vi "采水流程.vi"(10 "启动类型":enum16{"水样测试", "加标回收"}(ring), 11 "采配水参数":T1={"排空时间"=60.0, "润洗时间"=60.0, "进样超时时间"=300.0, "沉淀时间"=1800.0, "配水时间"=7200.0}) -> ()   [LabVIEW 2016, in "采配水.lvlib"]
panel:
  out "配水启动时间":timestamp
  in  "沉淀初始化":bool
  in  "配水初始化":bool
  in  "润洗初始化":bool
  in  "采样初始化":bool
  in  "排空初始化":bool
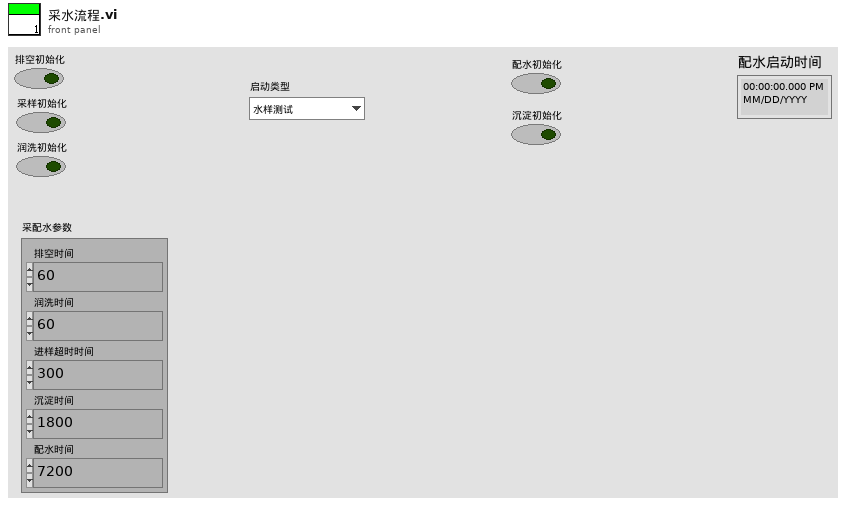
[diagram p1: front panel]
types:
  T1 = cluster{"排空时间":dbl, "润洗时间":dbl, "进样超时时间":dbl, "沉淀时间":dbl, "配水时间":dbl}
  T2 = typedef "采配水.lvlib/采配水流程.ctl" = u16
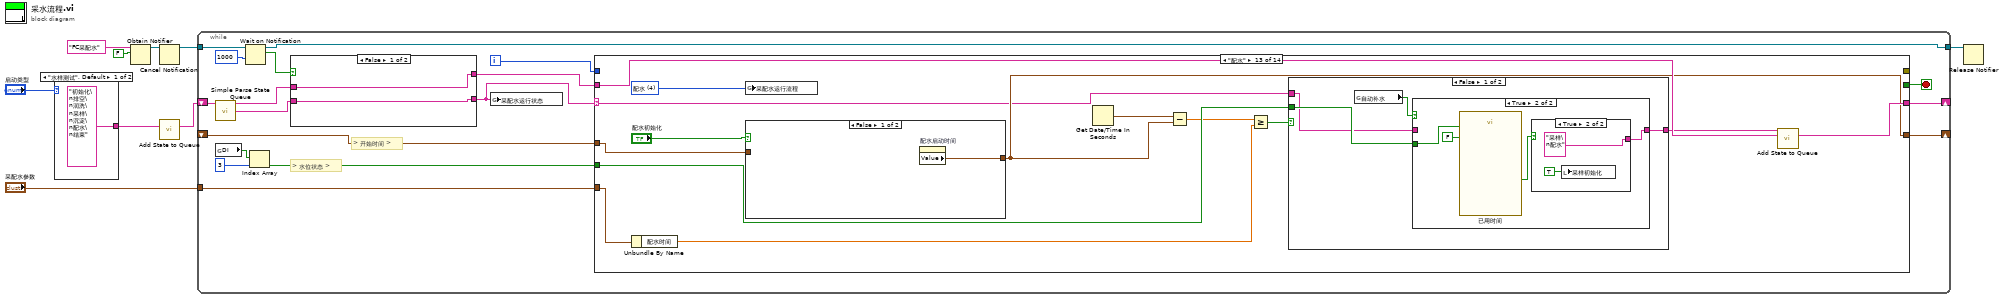
[diagram p0: block diagram]
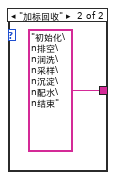
[diagram p2: hidden frame]
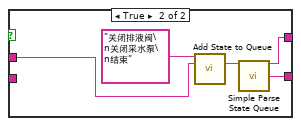
[diagram p3: hidden frame]
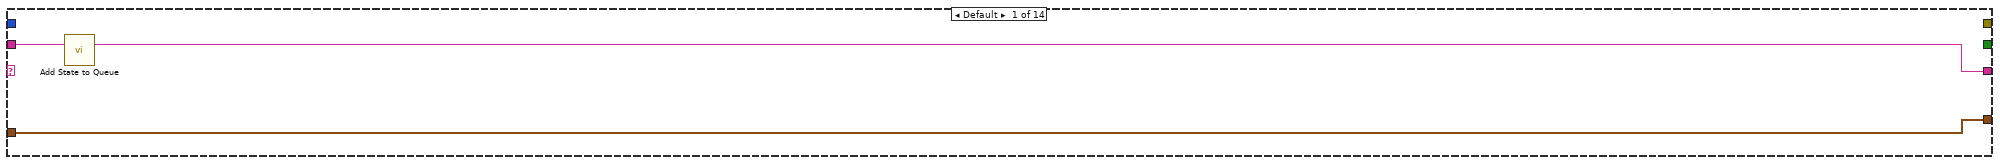
[diagram p4: hidden frame]
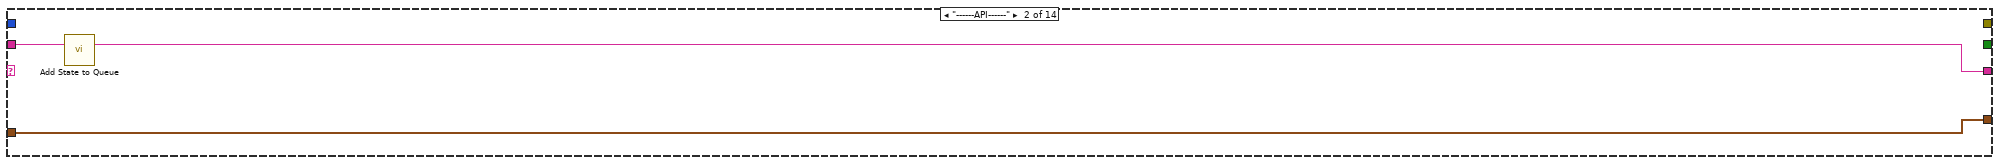
[diagram p5: hidden frame]
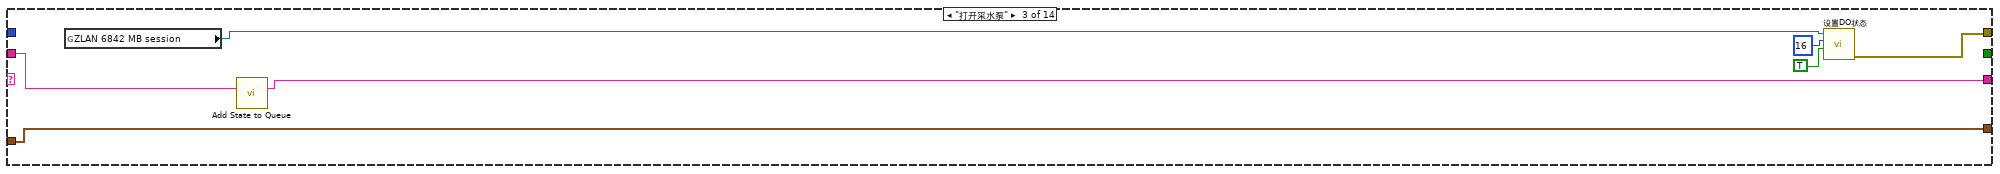
[diagram p6: hidden frame]
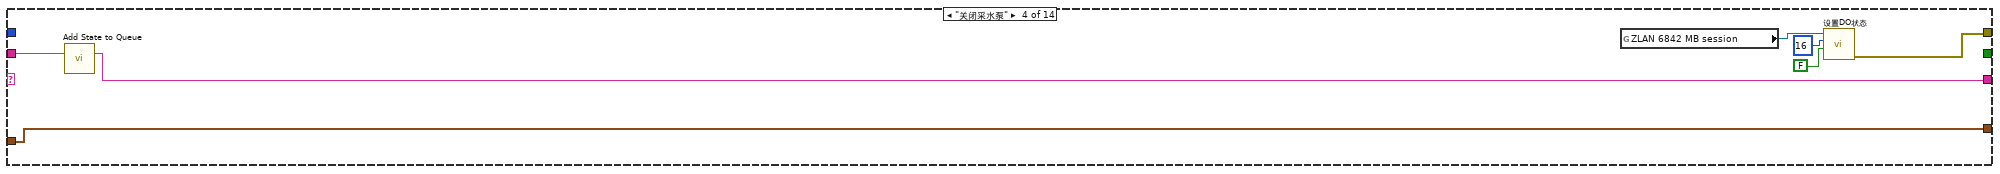
[diagram p7: hidden frame]
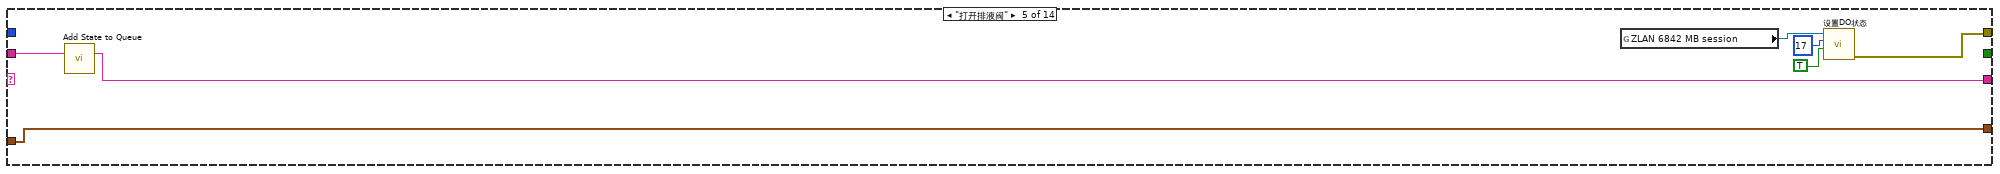
[diagram p8: hidden frame]
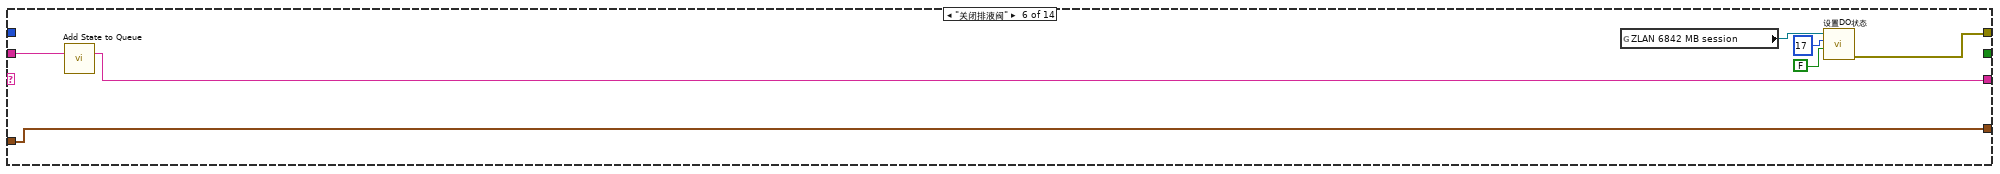
[diagram p9: hidden frame]
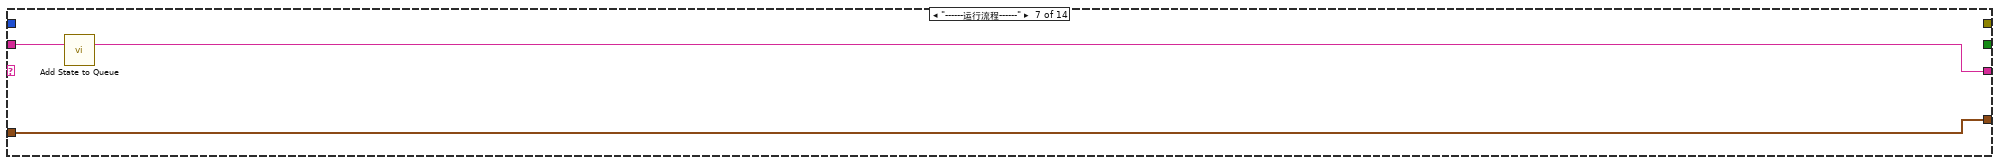
[diagram p10: hidden frame]
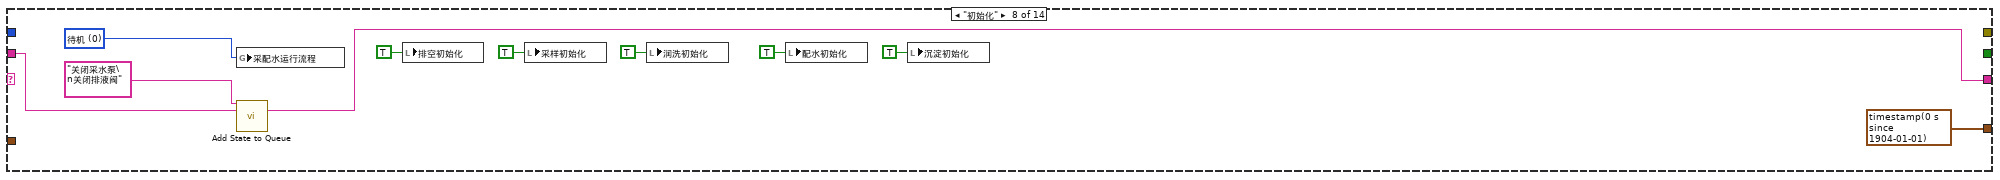
[diagram p11: hidden frame]
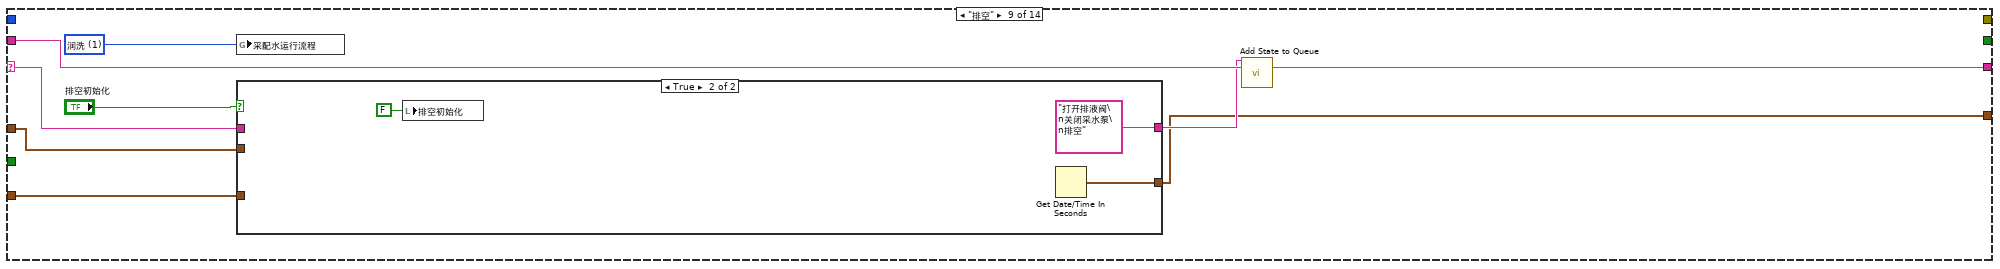
[diagram p12: hidden frame]
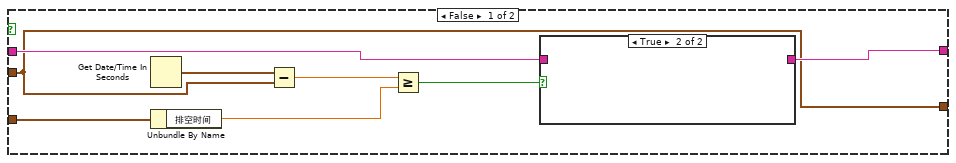
[diagram p13: hidden frame]
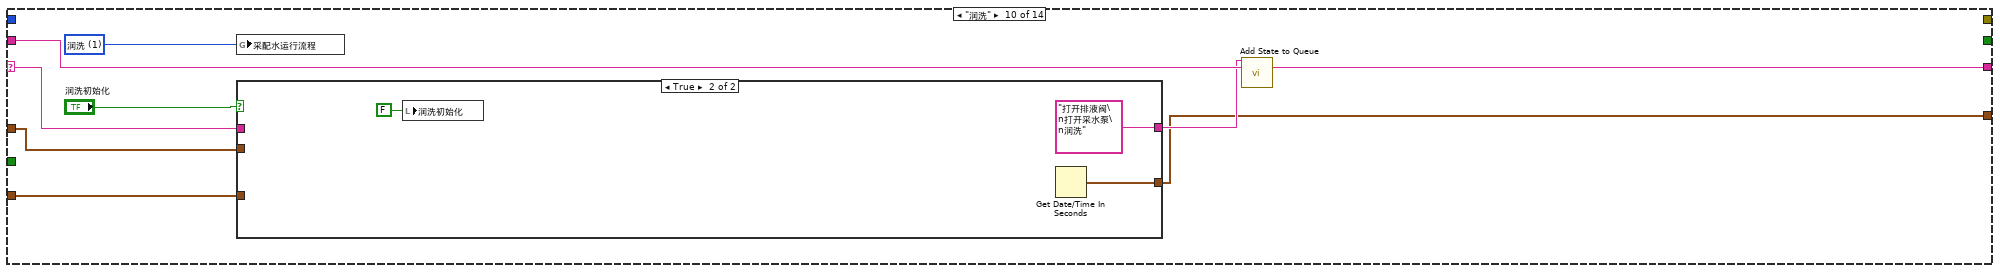
[diagram p15: hidden frame]
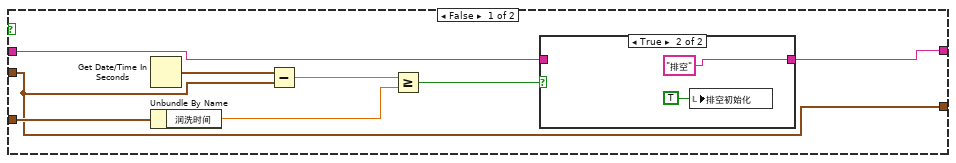
[diagram p16: hidden frame]
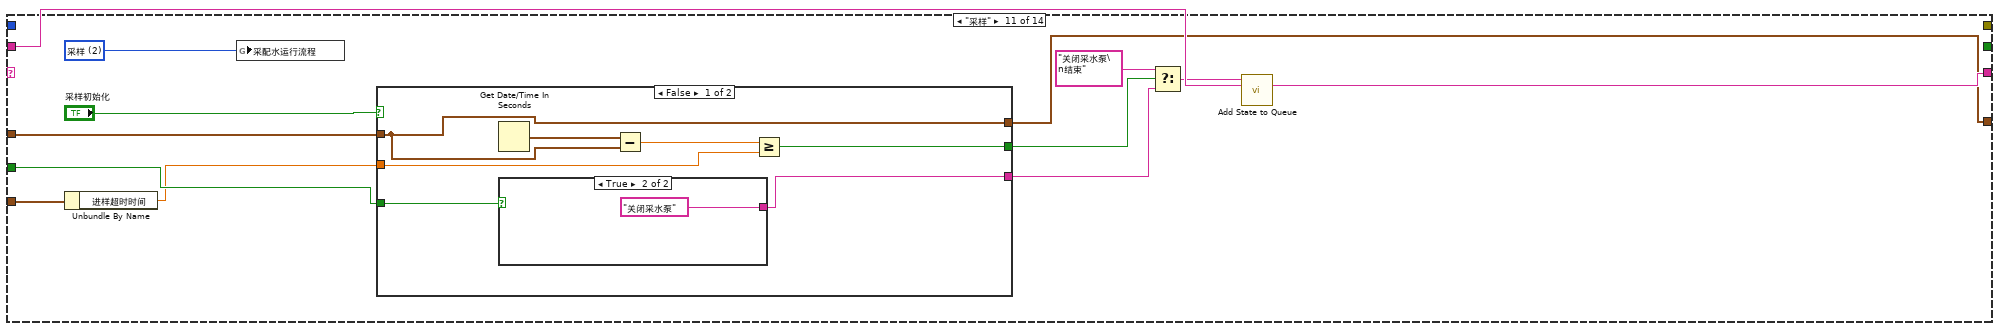
[diagram p18: hidden frame]
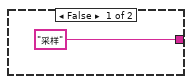
[diagram p19: hidden frame]
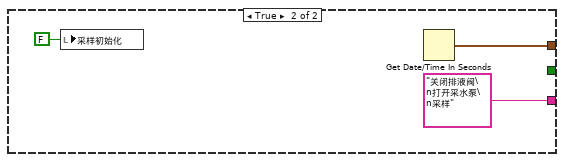
[diagram p20: hidden frame]
diagram:
  n1 = case shown="\"水样测试\", Default" "启动类型" {
    tunnel: ["初始化\n排空\n润洗\n采样\n沉淀\n配水\n结束" ("State(s) In (\"\")") "初始化\n排空\n润洗\n采样\n沉淀\n配水\n结束" ("State(s) In (\"\")")] -> w2
    frame "水样测试", Default {
    }
    frame "加标回收" {
    }
  }
  n2 = Obtain Notifier(name (unnamed)="FC采配水" ("名称（未命名）"), notification data type=FALSE) -> (notifier out=w6:refnum<notifier>)  [unwired: 2 in, 2 out]
  n3 = Cancel Notification(0:w6) -> (8:w5:refnum<notifier>)  [unwired: 1 in, 2 out]
  n4 = call "Add State to Queue.vi"("State(s) In (\"\")"=w2) -> ("States Out"=w9:string)  [unwired: 14 in]
  n5 = while {
    shift-right: [w28] -> _
    shift-left: w9 -> [w29]
    shift-right: [w27] -> _
    shift-left: _ -> [w26]
    tunnel: "采配水参数" -> [w21]
    tunnel: w5 -> [w20]
    tunnel: [w16] -> w4
    i -> [w12]
    stop <- w25 stop-if-true
    # "> 开始时间 >"
    # "> 水位状态 >"
    n6 = call "Simple Parse State Queue.vi"("State Queue"=w29) -> ("Remain States"=w15:string, "Next State"=w17:string)  [unwired: 13 in]
    n7 = global read "通讯全局变量.vi" "DI"() -> (w24:bool[])
    n8 = Wait on Notification(notifier=w20, timeout in ms (-1)=1000 ("超时毫秒(-1)")) -> (notifier out=w16:refnum<notifier>, notification=w18:bool)  [unwired: 2 in, 2 out]
    n9 = Index Array(array=w24, index=3 ("索引")) -> (element=w22:bool)
    n10 = case shown="False" w18 {
      tunnel: [w31 w33] -> w13
      tunnel: w17 -> [w31 _]
      tunnel: w15 -> [w30 w35]
      tunnel: [w30 w32] -> w14
      frame False {
      }
      frame True {
        n11 = call "Add State to Queue.vi"("State(s) In Front (\"\")"="关闭排液阀\n关闭采水泵\n结束" ("State(s) In (\"\")"), "State(s) In (\"\")"=w35) -> ("States Out"=w34:string)  [unwired: 13 in]
        n12 = call "Simple Parse State Queue.vi"("State Queue"=w34) -> ("Remain States"=w32:string, "Next State"=w33:string)  [unwired: 13 in]
      }
    }
    n13 = global write "通讯全局变量.vi" "采配水运行状态"(w13) -> ()
    n14 = case shown="\"配水\"" w13 {
      selector: w13 -> [_ _ _ _ _ _ _ _ w89 w109 _ w153 w170 w199]
      tunnel: w14 -> [w39 w42 w49 w56 w63 w70 w73 w83 w92 w111 w140 w160 w180 _]
      tunnel: [w38 w41 w48 w55 w62 w69 w72 w82 w91 w113 w139 w165 w183 w199] -> w28
      tunnel: w22 -> [_ _ _ _ _ _ _ _ _ _ w138 _ w182 _]
      tunnel: [_ _ w44 w51 w58 w65 _ _ _ _ _ _ _ _] -> _
      tunnel: [w37 w40 w43 w50 w57 w64 w71 timestamp(0 s since 1904-01-01) ("seconds since 1Jan1904") w84 w105 w128 w155 w174 w202] -> w27
      tunnel: w26 -> [w37 w40 w43 w50 w57 w64 w71 _ w90 w112 w133 w157 w176 w202]
      tunnel: [_ _ _ _ _ _ _ _ _ _ _ _ _ TRUE] -> w25
      tunnel: w21 -> [_ _ _ _ _ _ _ _ w86 w108 w137 w163 w179 _]
      tunnel: w12 -> [_ _ _ _ _ _ _ _ _ _ _ _ _ _]
      frame Default {
        n15 = call "Add State to Queue.vi"("State(s) In (\"\")"=w39) -> ("States Out"=w38:string)  [unwired: 14 in]
      }
      frame "------API------" {
        n16 = call "Add State to Queue.vi"("State(s) In (\"\")"=w42) -> ("States Out"=w41:string)  [unwired: 14 in]
      }
      frame "打开采水泵" {
        n17 = global read "通讯全局变量.vi" "ZLAN 6842 MB session"() -> (w45:refnum<class "MB_Master.lvclass">)
        n18 = call "Add State to Queue.vi"("State(s) In (\"\")"=w49) -> ("States Out"=w48:string)  [unwired: 14 in]
        n19 = call "设置DO状态.vi"("value"=TRUE, "address"=u16 16, "MB session in"=w45) -> ("error out"=w44:errorcluster)  [unwired: 7 in, 1 out]
      }
      frame "关闭采水泵" {
        n20 = call "Add State to Queue.vi"("State(s) In (\"\")"=w56) -> ("States Out"=w55:string)  [unwired: 14 in]
        n21 = global read "通讯全局变量.vi" "ZLAN 6842 MB session"() -> (w52:refnum<class "MB_Master.lvclass">)
        n22 = call "设置DO状态.vi"("value"=FALSE, "address"=u16 16, "MB session in"=w52) -> ("error out"=w51:errorcluster)  [unwired: 7 in, 1 out]
      }
      frame "打开排液阀" {
        n23 = call "Add State to Queue.vi"("State(s) In (\"\")"=w63) -> ("States Out"=w62:string)  [unwired: 14 in]
        n24 = global read "通讯全局变量.vi" "ZLAN 6842 MB session"() -> (w59:refnum<class "MB_Master.lvclass">)
        n25 = call "设置DO状态.vi"("value"=TRUE, "address"=u16 17, "MB session in"=w59) -> ("error out"=w58:errorcluster)  [unwired: 7 in, 1 out]
      }
      frame "关闭排液阀" {
        n26 = call "Add State to Queue.vi"("State(s) In (\"\")"=w70) -> ("States Out"=w69:string)  [unwired: 14 in]
        n27 = global read "通讯全局变量.vi" "ZLAN 6842 MB session"() -> (w66:refnum<class "MB_Master.lvclass">)
        n28 = call "设置DO状态.vi"("value"=FALSE, "address"=u16 17, "MB session in"=w66) -> ("error out"=w65:errorcluster)  [unwired: 7 in, 1 out]
      }
      frame "------运行流程------" {
        n29 = call "Add State to Queue.vi"("State(s) In (\"\")"=w73) -> ("States Out"=w72:string)  [unwired: 14 in]
      }
      frame "初始化" {
        w76 = T2 0 items=["待机", "润洗", "采样", "沉淀", "配水", "结束"] ("采配水运行流程")
        n30 = global write "通讯全局变量.vi" "采配水运行流程"(w76) -> ()
        n31 = call "Add State to Queue.vi"("State(s) In Front (\"\")"="关闭采水泵\n关闭排液阀" ("State(s) In Front (\"\")"), "State(s) In (\"\")"=w83) -> ("States Out"=w82:string)  [unwired: 13 in]
        n32 = local write "排空初始化"(TRUE ("排空初始化")) -> ()
        n33 = local write "采样初始化"(TRUE ("采样初始化")) -> ()
        n34 = local write "润洗初始化"(TRUE ("润洗初始化")) -> ()
        n35 = local write "配水初始化"(TRUE ("采样初始化")) -> ()
        n36 = local write "沉淀初始化"(TRUE ("润洗初始化")) -> ()
      }
      frame "排空" {
        w85 = T2 1 items=["待机", "润洗", "采样", "沉淀", "配水", "结束"] ("采配水运行流程")
        n37 = global write "通讯全局变量.vi" "采配水运行流程"(w85) -> ()
        n38 = case shown="True" "排空初始化" {
          tunnel: [w97 "打开排液阀\n关闭采水泵\n排空" ("State(s) In Front (\"\")")] -> w88
          tunnel: w90 -> [w93 _]
          tunnel: w89 -> [w96 _]
          tunnel: w86 -> [w95 _]
          tunnel: [w93 w102] -> w84
          frame False {
            n39 = Get Date/Time In Seconds() -> (seconds since 1Jan1904=w98:timestamp)
            n40 = Unbundle By Name(w95) -> ("排空时间"=w94:dbl)
            n41 = Subtract(x=w98, y=w93) -> (x-y=w99:dbl)
            n42 = Greater Or Equal?(x=w99, y=w94) -> (x >= y?=w100:bool)
            n43 = case shown="True" w100 {
              tunnel: [w101 _] -> w97
              tunnel: w96 -> [w101 _]
              frame False {
              }
              frame True {
              }
            }
          }
          frame True {
            n44 = local write "排空初始化"(FALSE ("排空初始化")) -> ()
            n45 = Get Date/Time In Seconds() -> (seconds since 1Jan1904=w102:timestamp)
          }
        }
        n46 = call "Add State to Queue.vi"("State(s) In Front (\"\")"=w88, "State(s) In (\"\")"=w92) -> ("States Out"=w91:string)  [unwired: 13 in]
      }
      frame "润洗" {
        w106 = T2 1 items=["待机", "润洗", "采样", "沉淀", "配水", "结束"] ("采配水运行流程")
        n47 = global write "通讯全局变量.vi" "采配水运行流程"(w106) -> ()
        n48 = case shown="True" "润洗初始化" {
          tunnel: [w118 "打开排液阀\n打开采水泵\n润洗" ("State(s) In Front (\"\")")] -> w110
          tunnel: w112 -> [w114 _]
          tunnel: w109 -> [w117 _]
          tunnel: w108 -> [w116 _]
          tunnel: [w114 w125] -> w105
          frame False {
            n49 = Get Date/Time In Seconds() -> (seconds since 1Jan1904=w119:timestamp)
            n50 = Unbundle By Name(w116) -> ("润洗时间"=w115:dbl)
            n51 = Subtract(x=w119, y=w114) -> (x-y=w120:dbl)
            n52 = Greater Or Equal?(x=w120, y=w115) -> (x >= y?=w121:bool)
            n53 = case shown="True" w121 {
              tunnel: [w122 "排空"] -> w118
              tunnel: w117 -> [w122 _]
              frame False {
              }
              frame True {
                n54 = local write "排空初始化"(TRUE ("排空初始化")) -> ()
              }
            }
          }
          frame True {
            n55 = local write "润洗初始化"(FALSE ("润洗初始化")) -> ()
            n56 = Get Date/Time In Seconds() -> (seconds since 1Jan1904=w125:timestamp)
          }
        }
        n57 = call "Add State to Queue.vi"("State(s) In Front (\"\")"=w110, "State(s) In (\"\")"=w111) -> ("States Out"=w113:string)  [unwired: 13 in]
      }
      frame "采样" {
        w129 = T2 2 items=["待机", "润洗", "采样", "沉淀", "配水", "结束"] ("采配水运行流程")
        n58 = Unbundle By Name(w137) -> ("进样超时时间"=w132:dbl)
        n59 = global write "通讯全局变量.vi" "采配水运行流程"(w129) -> ()
        n60 = case shown="False" "采样初始化" {
          tunnel: [w146 "关闭排液阀\n打开采水泵\n采样" ("State(s) In Front (\"\")")] -> w136
          tunnel: w138 -> [w147 _]
          tunnel: w133 -> [w141 _]
          tunnel: w132 -> [w143 _]
          tunnel: [w142 _] -> w131
          tunnel: [w141 w150] -> w128
          frame False {
            n61 = Get Date/Time In Seconds() -> (seconds since 1Jan1904=w144:timestamp)
            n62 = case shown="True" w147 {
              tunnel: ["采样" ("State(s) In Front (\"\")") "关闭采水泵" ("State(s) In Front (\"\")")] -> w146
              frame False {
              }
              frame True {
              }
            }
            n63 = Subtract(x=w144, y=w141) -> (x-y=w145:dbl)
            n64 = Greater Or Equal?(x=w145, y=w143) -> (x >= y?=w142:bool)
          }
          frame True {
            n65 = local write "采样初始化"(FALSE ("采样初始化")) -> ()
            n66 = Get Date/Time In Seconds() -> (seconds since 1Jan1904=w150:timestamp)
          }
        }
        n67 = Select(t="关闭采水泵\n结束" ("State(s) In Front (\"\")"), s=w131, f=w136) -> (s? t:f=w135:string)
        n68 = call "Add State to Queue.vi"("State(s) In Front (\"\")"=w135, "State(s) In (\"\")"=w140) -> ("States Out"=w139:string)  [unwired: 13 in]
      }
      frame "沉淀" {
        w164 = T2 3 items=["待机", "润洗", "采样", "沉淀", "配水", "结束"] ("采配水运行流程")
        n69 = Unbundle By Name(w163) -> ("沉淀时间"=w162:dbl)
        n70 = global write "通讯全局变量.vi" "采配水运行流程"(w164) -> ()
        n71 = case shown="True" "沉淀初始化" {
          tunnel: w157 -> [w166 _]
          tunnel: [w166 w167] -> w155
          frame False {
          }
          frame True {
            n72 = property on="沉淀初始化" class="Bool (严格)"("Value"=FALSE ("沉淀初始化")) -> ()  [unwired: 2 in, 2 out]
            n73 = Get Date/Time In Seconds() -> (seconds since 1Jan1904=w167:timestamp)
          }
        }
        n74 = Get Date/Time In Seconds() -> (seconds since 1Jan1904=w156:timestamp)
        n75 = Subtract(x=w156, y=w155) -> (x-y=w154:dbl)
        n76 = Greater Or Equal?(x=w154, y=w162) -> (x >= y?=w161:bool)
        n77 = case shown="False" w161 {
          tunnel: [w169 _] -> w159
          tunnel: w153 -> [w169 _]
          frame False {
          }
          frame True {
          }
        }
        n78 = call "Add State to Queue.vi"("State(s) In Front (\"\")"=w159, "State(s) In (\"\")"=w160) -> ("States Out"=w165:string)  [unwired: 13 in]
      }
      frame "配水" {
        w181 = T2 4 items=["待机", "润洗", "采样", "沉淀", "配水", "结束"] ("采配水运行流程")
        n79 = Unbundle By Name(w179) -> ("配水时间"=w172:dbl)
        n80 = global write "通讯全局变量.vi" "采配水运行流程"(w181) -> ()
        n81 = case shown="False" "配水初始化" {
          tunnel: w176 -> [_ _]
          tunnel: [w196 w198] -> w174
          frame False {
            n82 = property on="配水启动时间" class="AbsTime (严格)"() -> ("Value"=w196:timestamp)  [unwired: 2 in, 2 out]
          }
          frame True {
            n83 = Get Date/Time In Seconds() -> (seconds since 1Jan1904=w198:timestamp)
            "配水启动时间" <- w198
            n84 = property on="配水初始化" class="Bool (严格)"("Value"=FALSE ("配水初始化")) -> ()  [unwired: 2 in, 2 out]
          }
        }
        n85 = Get Date/Time In Seconds() -> (seconds since 1Jan1904=w175:timestamp)
        n86 = Subtract(x=w175, y=w174) -> (x-y=w173:dbl)
        n87 = Greater Or Equal?(x=w173, y=w172) -> (x >= y?=w171:bool)
        n88 = case shown="False" w171 {
          tunnel: w182 -> [w187 _]
          tunnel: w170 -> [w185 _]
          tunnel: [w184 _] -> w178
          frame False {
            n89 = global read "通讯全局变量断电保存.vi" "自动补水"() -> (w186:bool)
            n90 = case shown="True" w186 {
              tunnel: w187 -> [_ w191]
              tunnel: [w188 w189] -> w184
              tunnel: w185 -> [w188 _]
              frame False {
              }
              frame True {
                n91 = call "已用时间"("Reset"=w191, "Auto Reset"=FALSE) -> ("Time has Elapsed"=w190:bool)  [unwired: 10 in, 7 out]
                n92 = case shown="True" w190 {
                  tunnel: ["配水" ("State(s) In Front (\"\")") "采样\n配水" ("State(s) In Front (\"\")")] -> w189
                  frame False {
                  }
                  frame True {
                    n93 = local write "采样初始化"(TRUE ("采样初始化")) -> ()
                  }
                }
              }
            }
          }
          frame True {
          }
        }
        n94 = call "Add State to Queue.vi"("State(s) In Front (\"\")"=w178, "State(s) In (\"\")"=w180) -> ("States Out"=w183:string)  [unwired: 13 in]
      }
      frame "结束" {
        w200 = T2 0 items=["待机", "润洗", "采样", "沉淀", "配水", "结束"] ("采配水运行流程")
        n95 = global write "通讯全局变量.vi" "采配水运行流程"(w200) -> ()
      }
    }
  }
  n96 = Release Notifier(notifier=w4) -> ()  [unwired: 2 in, 3 out]
